vi "Reserve bitsequence.vi"(7 "Data in":i16[](array[numeric])=[0, 0, 0, 0], 13 "Reserve bitsequence":bool) -> (8 "Data out":i16[](array[numeric]))   [LabVIEW 2014]
panel:
  # "Copyright 2014 Vidrio Technologies\nScanImage 5 software is licensed under the Apache License, Version 2.0 (the \"License\"); you may not use any files contained\nwithin the ScanImage 5 release except in compliance with the License. You may obtain a copy of the License at\n http://www.apache.org/licenses/LICENSE-2.0\nUnless required by applicable law or agreed to in writing, software distributed under the License is distributed on an\n\"AS IS\" BASIS, WITHOUT WARRANTIES OR CONDITIONS OF ANY KIND, either express or implied. See the License for the\n specific language governing permissions and limitations under the License."
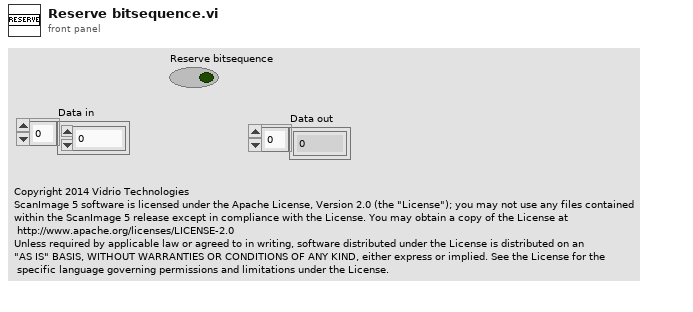
[diagram p1: front panel]
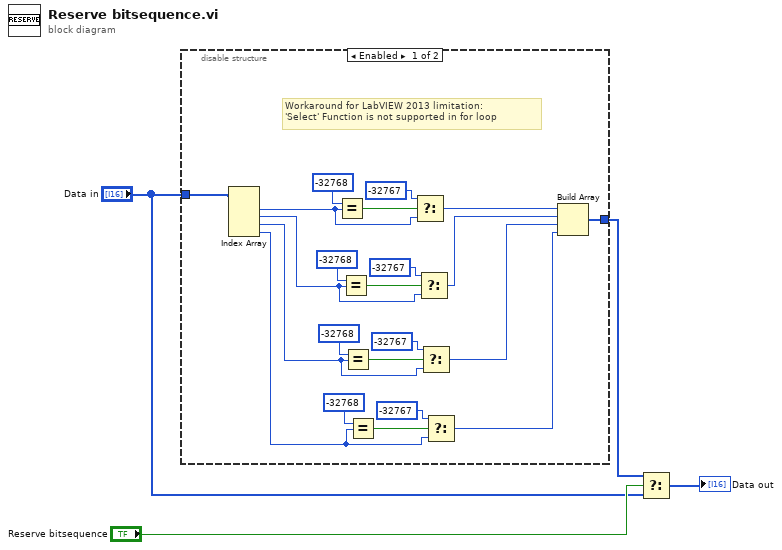
[diagram p0: block diagram]
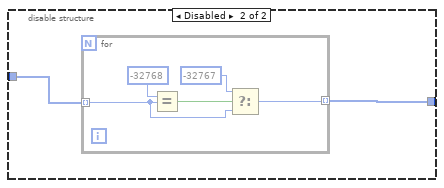
[diagram p2: hidden frame]
diagram:
  n1 = disable-structure shown="Enabled" {
    disable-tunnel: "Data in" -> [w23 w28]
    disable-tunnel: [w8 w27] -> w2
    frame Enabled {
      # "Workaround for LabVIEW 2013 limitation:\n'Select' Function is not supported in for loop"
      n2 = Index Array(array=w23) -> (element #1=w22:i16, element #2=w12:i16, element #3=w11:i16, element #4=w10:i16)  [unwired: 4 in]
      n3 = Equal?(x=i16 -32768, y=w22) -> (x = y?=w26:bool)
      n4 = Equal?(x=i16 -32768, y=w12) -> (x = y?=w20:bool)
      n5 = Equal?(x=i16 -32768, y=w11) -> (x = y?=w19:bool)
      n6 = Equal?(x=i16 -32768, y=w10) -> (x = y?=w16:bool)
      n7 = Select(t=i16 -32767, s=w26, f=w22) -> (s? t:f=w9:i16)
      n8 = Select(t=i16 -32767, s=w20, f=w12) -> (s? t:f=w7:i16)
      n9 = Select(t=i16 -32767, s=w19, f=w11) -> (s? t:f=w6:i16)
      n10 = Select(t=i16 -32767, s=w16, f=w10) -> (s? t:f=w5:i16)
      n11 = Build Array(w9, w7, w6, w5) -> (w8:i16[])
    }
    frame Disabled {
      n12 = for {
        tunnel: w28 -> [w30] mode=indexing
        tunnel: [w29] -> w27 mode=indexing
        n13 = Equal?(x=i16 -32768, y=w30) -> (x = y?=w33:bool)
        n14 = Select(t=i16 -32767, s=w33, f=w30) -> (s? t:f=w29:i16)
      }
    }
  }
  n15 = Select(t=w2, s="Reserve bitsequence", f="Data in") -> (s? t:f=→"Data out":i16[])
